vi "_FPGA_DeCycAdder.vi"(8 "DecycIncrement":u64, 9 "CurrentDecyc in":u64, 10 "TargetDecyc":u64, 11 "Direction":bool) -> (0 "ReachTarget":bool, 1 "CurrentDecyc out":u64)   [LabVIEW 2018]
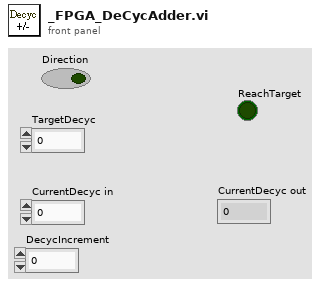
[diagram p1: front panel]
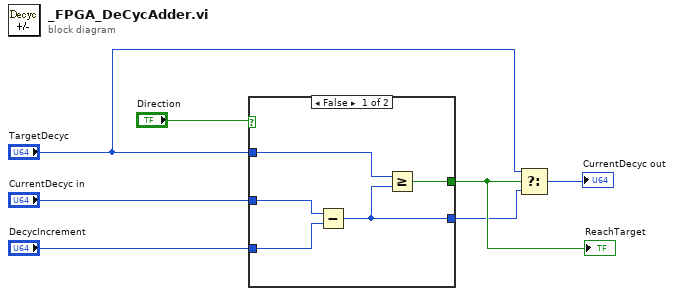
[diagram p0: block diagram]
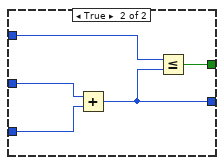
[diagram p2: hidden frame]
diagram:
  n1 = case shown="False" "Direction" {
    tunnel: "TargetDecyc" -> [w10 w15]
    tunnel: "CurrentDecyc in" -> [w12 w16]
    tunnel: "DecycIncrement" -> [w11 w17]
    tunnel: [w9 w14] -> w4
    tunnel: [w8 w13] -> w2
    frame False {
      n2 = Subtract(x=w12, y=w11) -> (x-y=w8:u64)
      n3 = Greater Or Equal?(x=w10, y=w8) -> (x >= y?=w9:bool)
    }
    frame True {
      n4 = Add(x=w16, y=w17) -> (x+y=w13:u64)
      n5 = Less Or Equal?(x=w15, y=w13) -> (x <= y?=w14:bool)
    }
  }
  "ReachTarget" <- w4
  n6 = Select(t="TargetDecyc", s=w4, f=w2) -> (s? t:f=→"CurrentDecyc out":u64)
